vi "spEVENTLOG Append Entry.vi"(8 "error in (no error)":errorcluster, 11 "Log Entry (\"\")":string) -> (0 "error out":errorcluster)   [LabVIEW 2011]
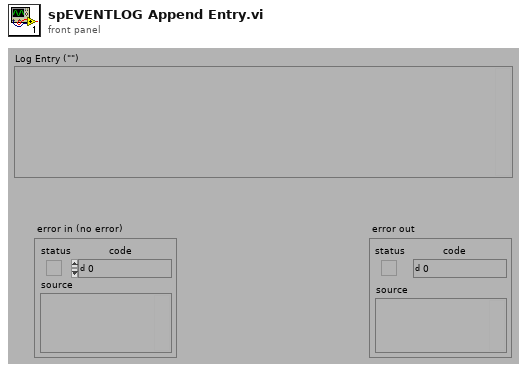
[diagram p1: front panel]
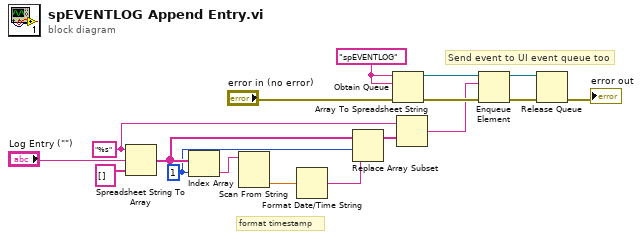
[diagram p0: block diagram]
diagram:
  w7 = 1 ("index")
  w5 = "%s" ("format string")
  w17 = "spEVENTLOG"
  # "format timestamp"
  # "Send event to UI event queue too"
  n1 = Spreadsheet String To Array(format string=w5, spreadsheet string="Log Entry (\"\")", array type (2D Dbl)=string[] []) -> (array=w9:string[])  [unwired: 1 in]
  n2 = Index Array(array=w9, index=w7) -> (element=w11:string)
  n3 = Scan From String(input string=w11) -> (output 1=w10:dbl)  [unwired: 4 in, 3 out]
  n4 = Format Date/Time String(seconds (now)=w10) -> (date/time string=w8:string)  [unwired: 2 in]
  n5 = Replace Array Subset(array=w9, new element=w8, index=w7) -> (w6:string[])
  n6 = Obtain Queue(name (unnamed)=w17, element data type=w17, error in (no error)="error in (no error)") -> (queue out=w16:refnum<queue>, error out=w15:errorcluster)  [unwired: 2 in, 1 out]
  n7 = Array To Spreadsheet String(array=w6, 3:w5) -> (spreadsheet string=w4:string)  [unwired: 1 in]
  n8 = Enqueue Element(queue=w16, element=w4, error in (no error)=w15) -> (queue out=w13:refnum<queue>, error out=w14:errorcluster)  [unwired: 1 in, 1 out]
  n9 = Release Queue(queue=w13, error in (no error)=w14) -> (error out=→"error out":errorcluster)  [unwired: 1 in, 2 out]
